vi "Destroy.vi"(8 "error in (no error)":errorcluster, 11 "CIF_Fifo_U8 in":refnum<class "CIF_Fifo_CAN_Multi.lvclass">) -> (0 "error out":errorcluster, 3 "CIF_Fifo_U8 out":refnum<class "CIF_Fifo_CAN_Multi.lvclass">)   [LabVIEW 2021]
uses:
  CIF_Fifo_CAN_Multi.lvclass
  D:/dev/Packages/Channel_Manager/src/CIFChannels/CIFChannels.lvclass
  CIFChannels/CIFChannels.lvclass/CIFChannels.ctl
  CIF_Fifo_CAN_Multi.lvclass/CIF_Fifo_CAN_Multi.ctl
  FIFO_U8/CIF_NIChn_Fifo_U8.lvclass
  FIFO_U8_Multi/CIF_Fifo_U8_Multi.lvclass
  CIFChannels/CIFChannels.lvclass
  D:/dev/Packages/Channel_Manager/src/CIF_NIChn/FIFO_U8_Multi/CIF_Fifo_U8_Multi.lvclass
  D:/dev/Packages/Channel_Manager/src/CIF_NIChn/FIFO_U8/CIF_NIChn_Fifo_U8.lvclass
  D:/dev/Packages/Channel_Manager/src/CIF_NIChn/NIChn/CIF_NIChn.lvclass
  D:/dev/Packages/Channel_Manager/src/CIF_NIChn/FIFO_CAN_Multi/CIF_Fifo_CAN_Multi.lvclass
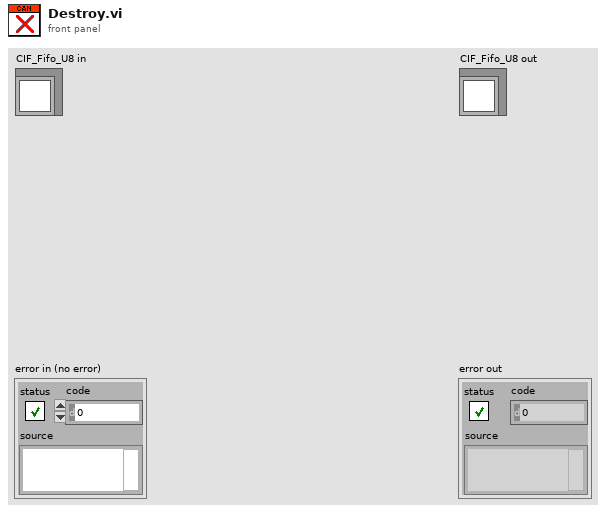
[diagram p1: front panel]
types:
  T1 = typedef "CIFChannels.lvclass/Direction.ctl" = enum16{"Publisher", "Subscriber"}
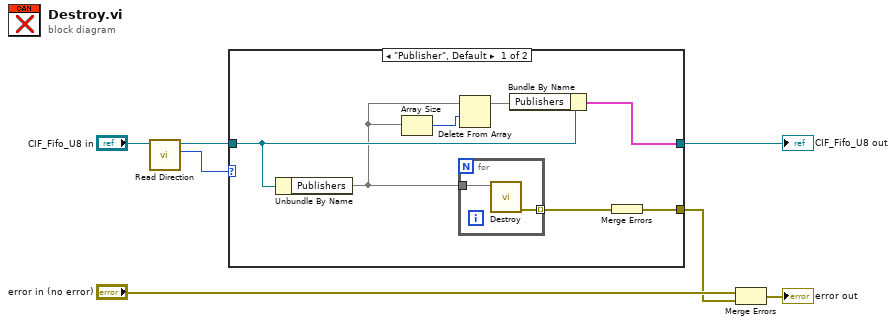
[diagram p0: block diagram]
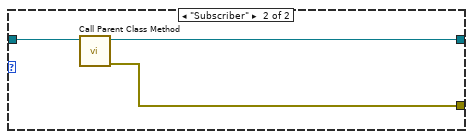
[diagram p2: hidden frame]
diagram:
  n1 = call "Read Direction.vi"("CIFChannels in"="CIF_Fifo_U8 in") -> ("Direction"=w6:T1, "CIFChannels out"=w5:refnum<class "CIF_Fifo_CAN_Multi.lvclass">)  [unwired: 8 in, 1 out]
  n2 = case shown="\"Publisher\", Default" w6 {
    tunnel: w5 -> [w14 w19]
    tunnel: [w11 w17] -> w2
    tunnel: [w13 w18] -> w4
    frame "Publisher", Default {
      n3 = Unbundle By Name(w14) -> ("Publishers"=w9)
      n4 = Array Size(array=w9) -> (size(s)=w10:i32)
      n5 = for {
        tunnel: w9 -> [w16]
        tunnel: [w15] -> w12 mode=indexing
        n6 = call-dynamic "Destroy.vi"("CIFFIFO in"=w16) -> ("error out"=w15:errorcluster)  [unwired: 9 in, 1 out]
      }
      n7 = Delete From Array(array=w9, length=w10) -> (array with subset deleted=w8)  [unwired: 1 in, 1 out]
      n8 = Bundle By Name(cluster=w14, "Publishers"=w8) -> (w13:cluster{})
      n9 = Merge Errors(w12) -> (w11:errorcluster)
    }
    frame "Subscriber" {
      n10 = call-parent "Call Parent Class Method"("CIF_Fifo_U8 in"=w19) -> ("error out"=w17:errorcluster, "CIF_Fifo_U8 out"=w18:refnum<class "CIF_Fifo_CAN_Multi.lvclass">)  [unwired: 9 in]
    }
  }
  "CIF_Fifo_U8 out" <- w4
  n11 = Merge Errors("error in (no error)", w2) -> (→"error out":errorcluster)
